vi "intToFloat.vi"(1 "bits":u16, 2 "x_min":fxp<+/-,32,17>, 3 "x_max":fxp<+/-,32,17>, 4 "x":u16 format="%x") -> (0 "Float":fxp<+/-,32,17>)   [LabVIEW 2019]
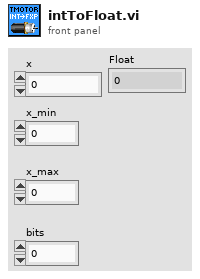
[diagram p1: front panel]
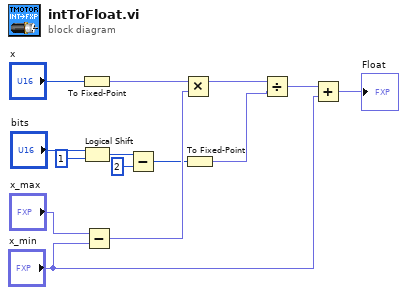
[diagram p0: block diagram]
diagram:
  n1 = To Fixed-Point(number="x") -> (fixed-point=w7:fxp<+/-,32,17>)  [unwired: 1 in]
  n2 = Logical Shift(y="bits", x=u32 1) -> (x << y=w11:u32)
  n3 = Subtract(x="x_max", y="x_min") -> (x-y=w8:fxp<+/-,32,17>)
  n4 = Subtract(x=w11, y=u32 2) -> (x-y=w6:u32)
  n5 = Multiply(x=w7, y=w8) -> (x*y=w4:fxp<+/-,64,32>)
  n6 = To Fixed-Point(number=w6) -> (fixed-point=w3:fxp<+/-,64,32>)  [unwired: 1 in]
  n7 = Divide(x=w4, y=w3) -> (x/y=w2:fxp<+/-,32,17>)
  n8 = Add(x=w2, y="x_min") -> (x+y=→"Float":fxp<+/-,32,17>)
